vi "Detect latest run.vi"(11 "Captures":path) -> (2 "Trigger new cloneable":bool, 3 "Capture path":path)   [LabVIEW 2026, in "Launcher.lvlib"]
uses:
  Launcher.lvlib
  <userlib>/_OpenG.lib/comparison/comparison.llb/Variant Changed__ogtk.vi
  <userlib>/_OpenG.lib/comparison/comparison.llb/openg_comparison__ogtk.lvlib
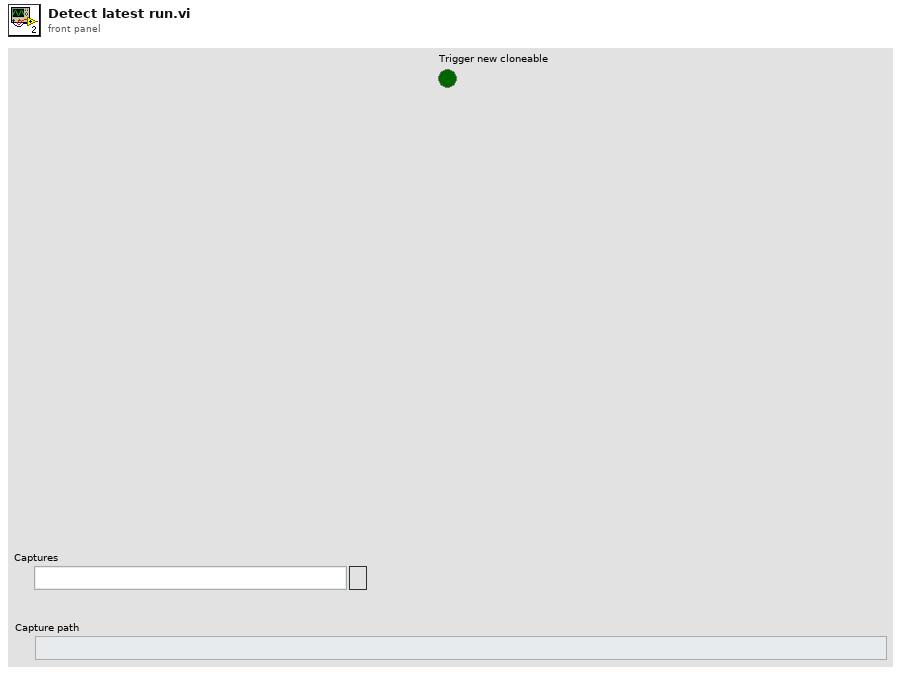
[diagram p1: front panel]
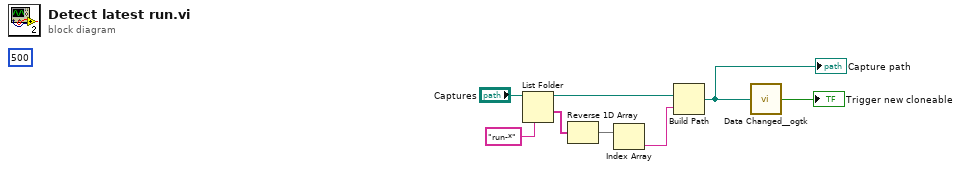
[diagram p0: block diagram]
diagram:
  (unwired) 500
  n1 = List Folder(path="Captures", pattern="run-*") -> (path out=w4:path, folder names=w3:string[])  [unwired: 2 in, 2 out]
  n2 = Reverse 1D Array(array=w3) -> (reversed array=w6:string[])
  n3 = Index Array(array=w6) -> (element=w7:string)  [unwired: 1 in]
  n4 = Build Path(base path=w4, name or relative path=w7) -> (appended path=w2:path)
  "Capture path" <- w2
  n5 = call-poly <userlib>:"Data Changed__ogtk.vi"("Variant"=w2) -> ("Changed"=→"Trigger new cloneable":bool)
